vi "Acquisition Message Loop.vi"(8 "error in (no error)":errorcluster, 9 "Data Queue":refnum<queue>, 10 "Data Notifier":refnum<notifier>, 11 "Message Queues":T1) -> (0 "error out":errorcluster)   [LabVIEW 2026, in "Acquisition.lvlib"]
doc: "Message loop for handling messages pertaining to the acquisition of data from the hardware."
uses:
  Acquisition.lvlib
  support/Message Queue/Message Queue.lvlib
  Controls/Acquisition State.ctl
  Support/Message Queue/Enqueue Message (Single).vi
  <vilib>/ErrorRing/Error Ring.xnode
  Controls/Vibration_Monitor_Config.ctl
  Controls/Vibration_Profile.ctl
  Controls/Options.ctl
  Controls/System_Settings.ctl
  Controls/Acquisition Metrics.ctl
  <vilib>/Utility/error.llb/Error Cluster From Error Code.vi
  Controls/Relay_Profile.ctl
  Controls/RPM_Profile.ctl
  Support/Message Queue/Message Cluster.ctl
  Support/Message Queue/All Message Queues.ctl
  Controls/Machine_State_Buffer.ctl
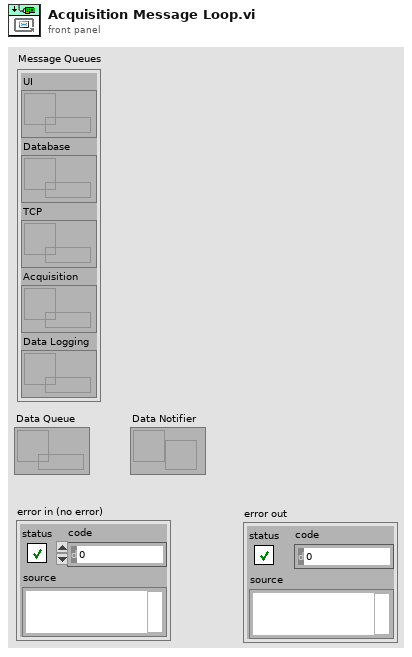
[diagram p1: front panel]
types:
  T1 = typedef "Message Queue.lvlib/All Message Queues.ctl" = cluster{"UI":refnum<queue>, "Database":refnum<queue>, "TCP":refnum<queue>, "Acquisition":refnum<queue>, "Data Logging":refnum<queue>}
  T2 = typedef "Acquisition.lvlib/Acquisition Metrics.ctl" = cluster{"Total_Samples":i64, "rpm":dbl}
  T3 = typedef "Vibration_Monitor_Config.ctl" = cluster{"Diagnostic_Modes":cluster{"Selected_Mode":string}, "Basic_Health":T4, "Complex_Machinery":T4, "Multi_Point":T4, "System_Settings":T5, "Relay":T7, "RPM":T8}
  T4 = typedef "Vibration_Profile.ctl" = cluster{"Task_Name":string, "Sample_Rate_Hz":dbl, "Samples_Per_Channel":i32, "RPM_PPR ":dbl}
  T5 = typedef "System_Settings.ctl" = cluster{"Simulation_Mode ":string, "Options":T6}
  T6 = typedef "Options.ctl" = enum16{"Healthy", "Unbalance_Alert", "Bearing_Fault_Critical", "Sweep_Test"}
  T7 = typedef "Relay_Profile.ctl" = cluster{"Task_Name":string}
  T8 = typedef "RPM_Profile.ctl" = cluster{"Task_Name":string, "Max_Expected_RPM":dbl, "Min_Expected_RPM":dbl, "Terminal_Name":string}
  T9 = typedef "Acquisition.lvlib/Acquisition State.ctl" = enum16{"Idle", "Acquiring"}
  T10 = typedef "Acquisition.lvlib/Hardware Configuration.ctl" = cluster{"Vibration_Task_Refnum":refnum<k21>, "Hardware_Fault_Status":errorcluster, "Trip_Relay_Task_Refnum":refnum<k21>, "RPM_Task_Refnum":refnum<k21>, "Is_Task_Running":bool}
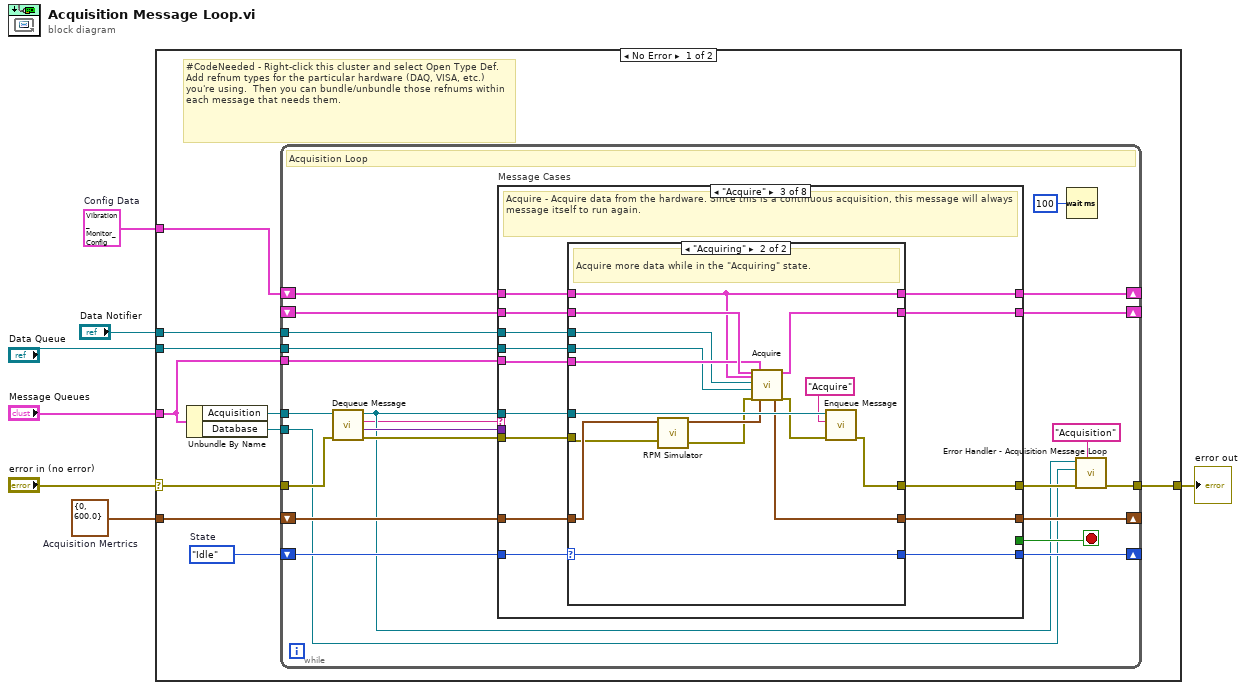
[diagram p0: block diagram]
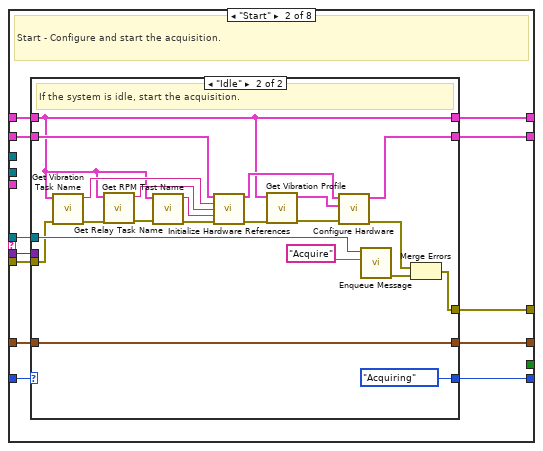
[diagram p3: hidden frame]
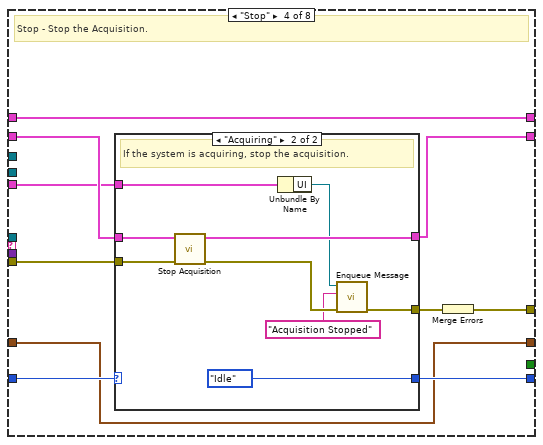
[diagram p6: hidden frame]
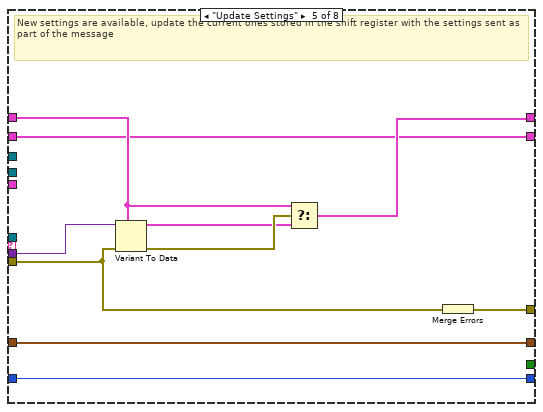
[diagram p8: hidden frame]
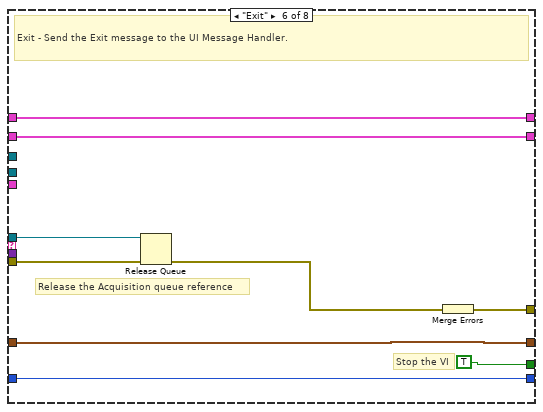
[diagram p9: hidden frame]
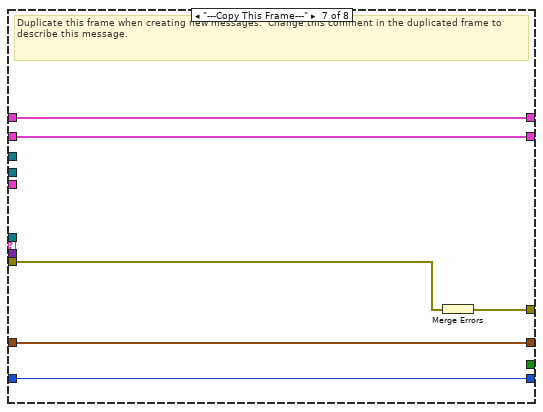
[diagram p10: hidden frame]
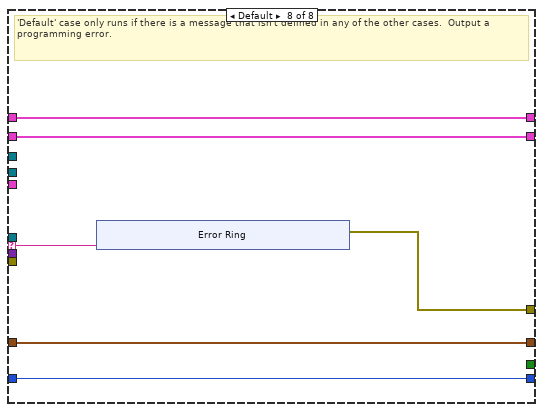
[diagram p11: hidden frame]
diagram:
  w1 = T2 {"Total_Samples"=0, "rpm"=600.0}  # Acquisition Mertrics
  w2 = T3 {"Diagnostic_Modes"={"Selected_Mode"=""}, "Basic_Health"={"Task_Name"="", "Sample_Rate_Hz"=0.0, "Samples_Per_Channel"=0, "RPM_PPR "=0.0}, "Complex_Machinery"={"Task_Name"="", "Sample_Rate_Hz"=0.0, "Samples_Per_Channel"=0, "RPM_PPR "=0.0}, "Multi_Point"={"Task_Name"="", "Sample_Rate_Hz"=0.0, "Samples_Per_Channel"=0, "RPM_PPR "=0.0}, "System_Settings"={"Simulation_Mode "="", "Options"=enum."Healthy"}, "Relay"={"Task_Name"="Local_Trip_Relay_Task"}, "RPM"={"Task_Name"="", "Max_Expected_RPM"=0.0, "Min_Expected_RPM"=0.0, "Terminal_Name"=""}}  # Config Data
  n1 = case shown="No Error" "error in (no error)" {
    selector: "error in (no error)" -> [w15 w179]
    tunnel: "Message Queues" -> [w9 _]
    tunnel: [w16 w179] -> w6
    tunnel: "Data Notifier" -> [w14 _]
    tunnel: "Data Queue" -> [w13 _]
    tunnel: w2 -> [w11 _]
    tunnel: w1 -> [w10 _]
    frame No Error {
      w12 = Acquisition_State."Idle"  # State
      # "#CodeNeeded - Right-click this cluster and select Open Type Def.  Add refnum types for the particular hardware (DAQ, VISA, etc.) you're using.  Then you can bundle/unbundle those refnums within each message that needs them."
      n2 = Unbundle By Name(w9) -> ("Acquisition"=w17:refnum<queue>, "Database"=w8:refnum<queue>)
      n3 = while {
        tunnel: w17 -> [w34]
        shift-right: [w39] -> _
        shift-left: w11 -> [w40]
        tunnel: w14 -> [w33]
        tunnel: w13 -> [w32]
        shift-right: [w30] -> _
        shift-left: w12 -> [w31]
        tunnel: w15 -> [w37]
        tunnel: [w29] -> w16
        shift-right: [w27] -> _
        shift-left: _ -> [w26]
        shift-right: [w23] -> _
        shift-left: w10 -> [w25]
        tunnel: w9 -> [w21]
        tunnel: w8 -> [w20]
        stop <- w38 stop-if-true
        # "Acquisition Loop"
        n4 = call "Dequeue Message.vi"("error in (no error)"=w37, "Message Queue"=w34) -> ("error out"=w36:errorcluster, "Message Data"=w35:variant, "Message"=w18:string, "dup Message Queue"=w22:refnum<queue>)  [unwired: 6 in]
        n5 = case "Message Cases" shown="\"Acquire\"" w18 {
          selector: w18 -> [_ _ _ _ _ _ _ w168]
          tunnel: w22 -> [_ w54 w96 _ _ w154 _ _]
          tunnel: w36 -> [w41 w55 w95 w127 w144 w156 w165 _]
          tunnel: [w41 w57 w97 w128 w150 w158 w163 w169] -> w28
          tunnel: w40 -> [w45 w56 w93 w125 w146 w157 w164 w171]
          tunnel: [w45 w53 w94 w125 w145 w157 w164 w171] -> w39
          tunnel: [_ _ _ _ _ TRUE _ _] -> w38
          tunnel: w35 -> [_ w50 _ _ w149 _ _ _]
          tunnel: w33 -> [_ _ w92 _ _ _ _ _]
          tunnel: w32 -> [_ _ w91 _ _ _ _ _]
          tunnel: w31 -> [w44 w51 w89 w124 w143 w153 w162 w170]
          tunnel: [w44 w52 w90 w123 w143 w153 w162 w170] -> w30
          tunnel: [w43 w49 w87 w121 w142 w152 w161 w167] -> w27
          tunnel: w26 -> [w43 w48 w88 w122 w142 w152 w161 w167]
          tunnel: w25 -> [w42 w47 w86 w120 w141 w151 w160 w166]
          tunnel: [w42 w46 w85 w120 w141 w151 w160 w166] -> w23
          tunnel: w21 -> [_ _ w84 w119 _ _ _ _]
          frame "Initialize" {
            # "Initialize  - Initialize is currently a no-op.  The hardware initialization takes place in the 'Start' message."
          }
          frame "Start" {
            # "Start - Configure and start the acquisition."
            n6 = case shown="\"Idle\"" w51 {
              selector: w51 -> [w60 _]
              tunnel: [w61 w83] -> w57
              tunnel: w56 -> [w62 w64]
              tunnel: w55 -> [w61 w77]
              tunnel: w54 -> [_ w78]
              tunnel: [w62 w64] -> w53
              tunnel: [w60 Acquisition_State."Acquiring" ("Acquisition State")] -> w52
              tunnel: w50 -> [_ _]
              tunnel: [w59 w72] -> w49
              tunnel: w48 -> [w59 w71]
              tunnel: w47 -> [w58 w70]
              tunnel: [w58 w70] -> w46
              frame "Acquiring" {
                # "The system is already acquiring. Ignore the \"Start\" message."
              }
              frame "Idle" {
                # "If the system is idle, start the acquisition."
                n7 = call "Get Vibration Task Name.vi"("error in (no error)"=w77, "Config Data"=w64) -> ("error out"=w69:errorcluster, "Active Task Name"=w68:string)  [unwired: 8 in]
                n8 = call "Get Relay Task Name.vi"("error in (no error)"=w69, "Config Data"=w64) -> ("error out"=w66:errorcluster, "Relay Task Name"=w67:string)  [unwired: 8 in]
                n9 = call "Get RPM Tast Name.vi"("error in (no error)"=w66, "Config Data"=w64) -> ("error out"=w65:errorcluster, "RPM Task Name"=w63:string)  [unwired: 8 in]
                n10 = call "Initialize Hardware References.vi"("Hardware Resources in"=w71, "Vibration Task Name"=w68, "Relay Task Name"=w67, "RPM Task Name"=w63, "error in (no error)"=w65) -> ("Hardware Resources out"=w73:T10, "error out"=w75:errorcluster)  [unwired: 9 in]
                n11 = call "Get Vibration Profile.vi"("error in (no error)"=w75, "Config Data"=w64) -> ("error out"=w74:errorcluster, "Active Vibration Profile"=w76:T4)  [unwired: 8 in]
                n12 = call "Configure Hardware.vi"("error in (no error)"=w74, "Active_Profile"=w76, "Hardware Resources in"=w73) -> ("error out"=w81:errorcluster, "Hardware Resources out"=w72:T10)  [unwired: 7 in]
                n13 = call-poly "Enqueue Message.vi"("Message"="Acquire", "Message Queue"=w78) -> ("error out"=w82:errorcluster)  [unwired: 8 in, 1 out]
                n14 = Merge Errors(w81, w82) -> (w83:errorcluster)
              }
            }
          }
          frame "Acquire" {
            # "Acquire - Acquire data from the hardware. Since this is a continuous acquisition, this message will always message itself to run again."
            n15 = case shown="\"Acquiring\"" w89 {
              selector: w89 -> [w100 w116]
              tunnel: [w101 w107] -> w97
              tunnel: w96 -> [_ w118]
              tunnel: w95 -> [w101 w104]
              tunnel: [w102 w111] -> w94
              tunnel: w93 -> [w102 w111]
              tunnel: w92 -> [_ w110]
              tunnel: w91 -> [_ w109]
              tunnel: [w100 w116] -> w90
              tunnel: w88 -> [w99 w115]
              tunnel: [w99 w114] -> w87
              tunnel: w86 -> [w98 w105]
              tunnel: [w98 w113] -> w85
              tunnel: w84 -> [_ w112]
              frame "Idle" {
                # "Ignore \"Acquire\" messages when the acquisition is idle."
              }
              frame "Acquiring" {
                # "Acquire more data while in the \"Acquiring\" state."
                n16 = call "RPM Simulator.vi"("error in (no error)"=w104, "Acquisition Mertrics in"=w105) -> ("error out"=w103:errorcluster, "Acquisition Mertrics out"=w106:T2)  [unwired: 8 in]
                n17 = call "Acquire.vi"("Hardware Resources in"=w115, "Config Data"=w111, "Data Notifier"=w110, "Data Queue"=w109, "error in (no error)"=w103, "Message Queues"=w112, "Acquisition Metrics in"=w106) -> ("Acquisition Metrics out"=w113:T2, "Hardware Resources out"=w114:T10, "error out"=w108:errorcluster)  [unwired: 10 in]
                n18 = call-poly "Enqueue Message.vi"("error in (no error)"=w108, "Message"="Acquire", "Message Queue"=w118) -> ("error out"=w107:errorcluster)  [unwired: 7 in, 1 out]
              }
            }
          }
          frame "Stop" {
            # "Stop - Stop the Acquisition."
            n19 = case shown="\"Acquiring\"" w124 {
              selector: w124 -> [w130 _]
              tunnel: w127 -> [w131 w140]
              tunnel: [w131 w137] -> w126
              tunnel: [w130 Acquisition_State."Idle" ("State")] -> w123
              tunnel: w122 -> [w129 w135]
              tunnel: [w129 w134] -> w121
              tunnel: w119 -> [_ w133]
              frame "Idle" {
                # "The system is already idle. Ignore the \"Stop\" message."
              }
              frame "Acquiring" {
                # "If the system is acquiring, stop the acquisition."
                n20 = call "Stop Acquisition.vi"("error in (no error)"=w140, "Hardware Resources in"=w135) -> ("error out"=w139:errorcluster, "Hardware Resources out"=w134:T10)  [unwired: 8 in]
                n21 = Unbundle By Name(w133) -> ("UI"=w132:refnum<queue>)
                n22 = call-poly "Enqueue Message.vi"("error in (no error)"=w139, "Message"="Acquisition Stopped", "Message Queue"=w132) -> ("error out"=w137:errorcluster)  [unwired: 7 in, 1 out]
              }
            }
            n23 = Merge Errors(w126) -> (w128:errorcluster)
          }
          frame "Update Settings" {
            # "New settings are available, update the current ones stored in the shift register with the settings sent as part of the message"
            n24 = Variant To Data(error in=w144, type=w146, Variant=w149) -> (data=w147:T3, error out=w148:errorcluster)
            n25 = Select(t=w146, s=w148, f=w147) -> (s? t:f=w145:T3)
            n26 = Merge Errors(w144) -> (w150:errorcluster)
          }
          frame "Exit" {
            # "Release the Acquisition queue reference"
            # "Stop the VI"
            # "Exit - Send the Exit message to the UI Message Handler."
            n27 = Release Queue(queue=w154, error in (no error)=w156) -> (error out=w155:errorcluster)  [unwired: 1 in, 2 out]
            n28 = Merge Errors(w155) -> (w158:errorcluster)
          }
          frame "---Copy This Frame---" {
            # "Duplicate this frame when creating new messages.  Change this comment in the duplicated frame to describe this message."
            n29 = Merge Errors(w165) -> (w163:errorcluster)
          }
          frame Default {
            # "'Default' case only runs if there is a message that isn't defined in any of the other cases.  Output a programming error."
            n30 = xnode "Error Ring"("parameter 0"=w168) -> ("error out"=w169:errorcluster)
          }
        }
        n31 = Wait (ms)(milliseconds to wait=u32 100) -> ()  [unwired: 1 out]
        n32 = call "Error Handler - Acquisition Message Loop.vi"("Loop"="Acquisition", "error in (no error)"=w28, "Database"=w20, "Message Queue"=w22) -> ("dup error in"=w29:errorcluster)  [unwired: 6 in, 1 out]
      }
    }
    frame Error {
    }
  }
  "error out" <- w6
